vi "Enqueue - Acquire Command.vi"(7 "Insert?":bool=TRUE caption="Insert? (T)", 8 "error in (no error)":errorcluster, 9 "Data":T1=variant(string "Default"), 10 "Command":string, 11 "Queue in":T2) -> (0 "error out":errorcluster, 3 "Queue Out (dup)":T2)   [LabVIEW 2010]
doc: "This VI inserts a command into the queue appending \"Acquire - \" to the Command field, with variant data.\n\nInputs:\nQueue in - queue reference (queue is cluster of Command (str) and Data (variant))\nCommand - (str) command to append to \"Acquire - \" and insert into queue\nData - (variant) data to insert with command into queue\nInsert? - (bool) allows logic to be connected to determine if item should be inserted into the queue or skipped\nerror in - error input cluster\n\nOutputs:\nQueue out (dup) - duplicate of input queue reference\nerror out - error output cluster"
uses:
  <userlib>/Common/Queue with Cluster/TYP_Queue with Cluster Reference.ctl
  Controls/TYP_VariantDefault.ctl
  UserDefined Command class/UserDefined Command class.lvclass
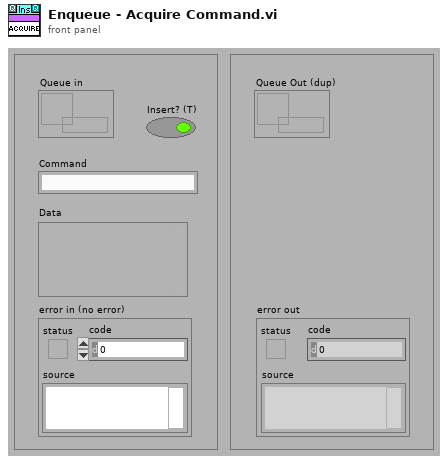
[diagram p1: front panel]
types:
  T1 = typedef "TYP_VariantDefault.ctl" = variant
  T2 = typedef "TYP_Queue with Cluster Reference.ctl" = refnum<queue>
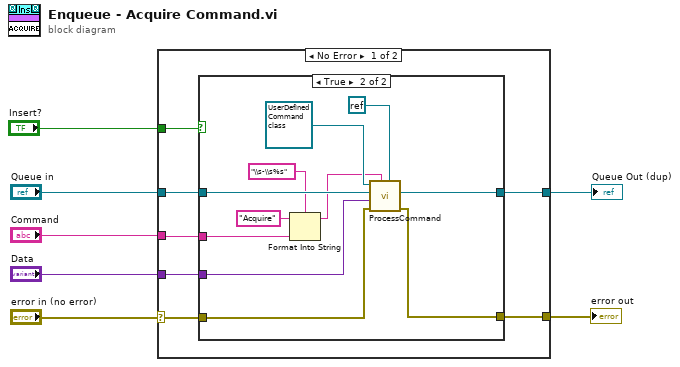
[diagram p0: block diagram]
diagram:
  n1 = case shown="No Error" "error in (no error)" {
    selector: "error in (no error)" -> [w10 w28]
    tunnel: "Queue in" -> [w14 w29]
    tunnel: [w13 w29] -> w6
    tunnel: "Data" -> [w12 _]
    tunnel: "Command" -> [w9 _]
    tunnel: [w11 w28] -> w3
    tunnel: "Insert?" -> [w8 _]
    frame No Error {
      n2 = case shown="True" w8 {
        tunnel: w14 -> [w16 w27]
        tunnel: [w16 w26] -> w13
        tunnel: w12 -> [_ w25]
        tunnel: [w15 w24] -> w11
        tunnel: w10 -> [w15 w23]
        tunnel: w9 -> [_ w20]
        frame False {
        }
        frame True {
          n3 = Format Into String(format string="\\s-\\s%s", initial string="Acquire", w20) -> (resulting string=w19:string)  [unwired: 1 in, 1 out]
          n4 = call-dynamic "ProcessCommand.vi"("Ctl Refnum"=refnum<k0> refnum, "Command"=w19, "error in (no error)"=w23, "Data"=w25, "Queue with Cluster Reference"=w27, "UserDefined Command class in"=refnum<class "UserDefined Command class.lvclass"> refnum) -> ("error out"=w24:errorcluster, "Queue (dup)"=w26:T2)  [unwired: 3 in, 1 out]
        }
      }
    }
    frame Error {
    }
  }
  "Queue Out (dup)" <- w6
  "error out" <- w3
